vi "Read Registers.vi"(0 "RS485 reference":refnum<class "Modbus Master.lvclass">, 1 "Number of inputs":u16, 2 "Starting address":u16, 3 "Serial reference":refnum<visa-resource-name>, 4 "Serial?":bool, 5 "error in":errorcluster) -> (14 "RS485 out":refnum<class "Modbus Master.lvclass">, 15 "register values":u16[](array[numeric]), 17 "Serial reference out":refnum<visa-resource-name>, 19 "error out":errorcluster)   [LabVIEW 2023]
uses:
  <vilib>/NI/Modbus Library/API/Master/Modbus Master.lvclass
  RS485/RS485.lvlib
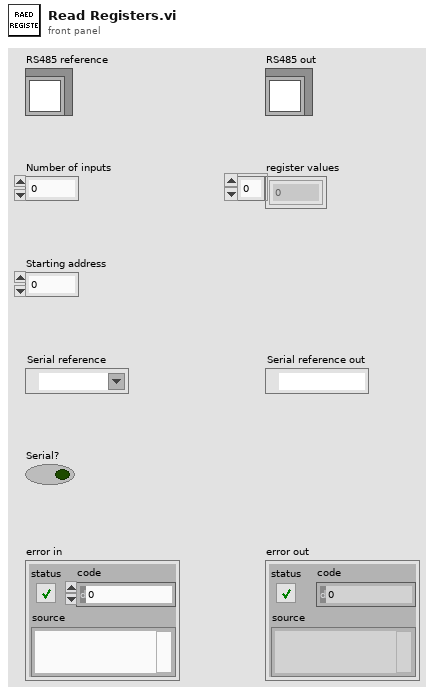
[diagram p1: front panel]
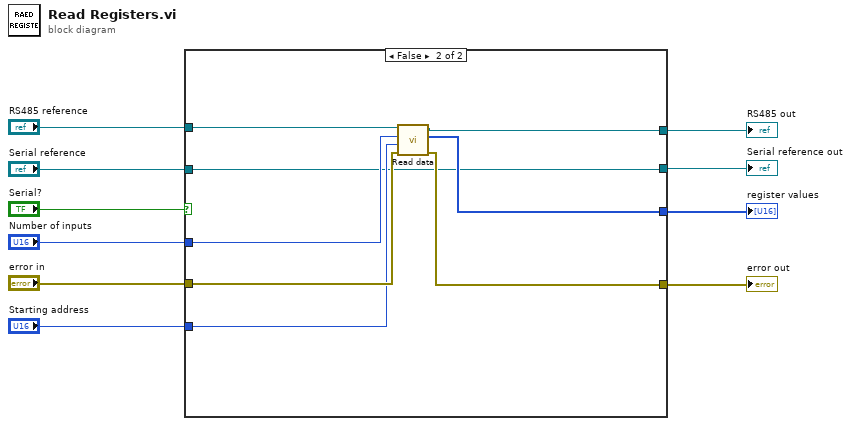
[diagram p0: block diagram]
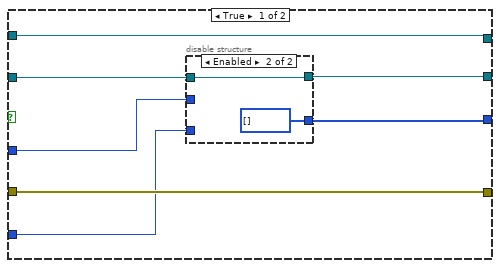
[diagram p2: hidden frame]
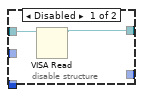
[diagram p3: hidden frame]
diagram:
  n1 = case shown="False" "Serial?" {
    tunnel: "RS485 reference" -> [w16 w29]
    tunnel: "Serial reference" -> [w17 w22]
    tunnel: "error in" -> [w14 w28]
    tunnel: "Number of inputs" -> [w13 w27]
    tunnel: "Starting address" -> [w12 w26]
    tunnel: [w16 w25] -> w4
    tunnel: [w11 w24] -> w3
    tunnel: [w14 w23] -> w2
    tunnel: [w15 w22] -> w1
    frame True {
      n2 = disable-structure shown="Enabled" {
        disable-tunnel: w17 -> [w19 w21]
        disable-tunnel: [w18 w21] -> w15
        disable-tunnel: w13 -> [_ _]
        disable-tunnel: w12 -> [_ _]
        disable-tunnel: [_ u16[] [] ("register values")] -> w11
        frame Disabled {
          n3 = VISA Read(VISA resource name=w19) -> (VISA resource name out=w18:refnum<visa-resource-name>)  [unwired: 2 in, 3 out]
        }
        frame Enabled {
        }
      }
    }
    frame False {
      n4 = call "Read data.vi"("error in"=w28, "starting address"=w26, "number of inputs"=w27, "Modbus master in"=w29) -> ("error out"=w23:errorcluster, "register values"=w24:u16[], "Modbus master out"=w25:refnum<class "Modbus Master.lvclass">)  [unwired: 5 in]
    }
  }
  "RS485 out" <- w4
  "register values" <- w3
  "error out" <- w2
  "Serial reference out" <- w1
